vi "Configure Receiver Leveling Sweep Safe Mode.vi"(4 "Safe Mode Maximum Power Level (30)":dbl=30.0, 5 "Maximum Step Power Level (0)":dbl, 6 "Safe Mode Minimum Power Level (-200)":dbl=-200.0, 7 "Enable Safe Mode (F: Disabled)":bool, 8 "error in (no error)":errorcluster, 9 "Port ( 1)":i32=1, 10 "Channel (1)":i32=1, 11 "VISA resource name":refnum<visa-resource-name>) -> (0 "error out":errorcluster, 3 "VISA resource name out":refnum<visa-resource-name>)   [LabVIEW 2022 SP3, in "Agilent ENA Series.lvlib"]
doc: "Configures the receiver leveling information while in safe mode.\n\nNote:\nValid for E5072A only."
uses:
  Agilent ENA Series.lvlib
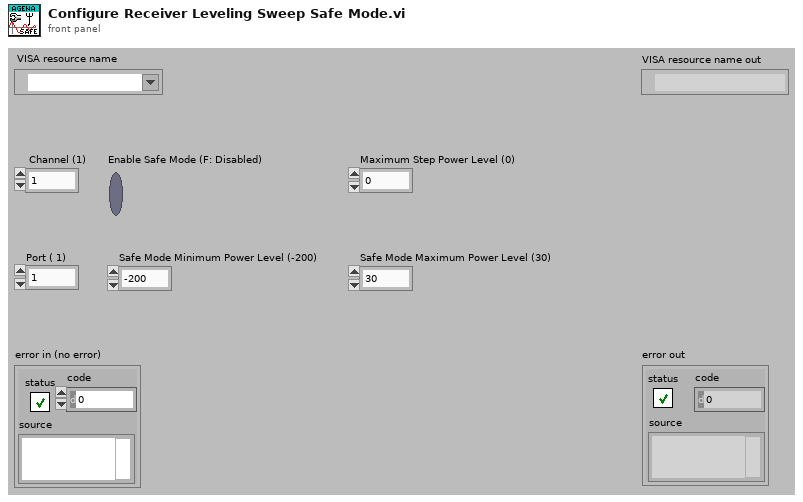
[diagram p1: front panel]
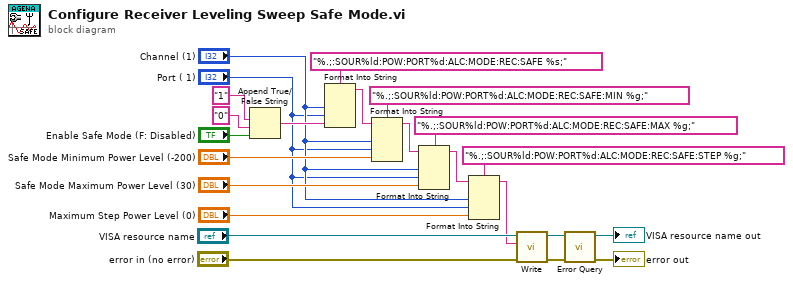
[diagram p0: block diagram]
diagram:
  n1 = Append True/False String(1:"Enable Safe Mode (F: Disabled)", 2:"0" ("false string"), 3:"1" ("true string")) -> (0:w16:string)  [unwired: 1 in]
  n2 = Format Into String(format string="%.;:SOUR%ld:POW:PORT%d:ALC:MODE:REC:SAFE %s;", "Channel (1)", "Port ( 1)", w16) -> (resulting string=w3:string)  [unwired: 2 in, 1 out]
  n3 = Format Into String(format string="%.;:SOUR%ld:POW:PORT%d:ALC:MODE:REC:SAFE:MIN %g;", initial string=w3, "Channel (1)", "Port ( 1)", "Safe Mode Minimum Power Level (-200)") -> (resulting string=w2:string)  [unwired: 1 in, 1 out]
  n4 = Format Into String(format string="%.;:SOUR%ld:POW:PORT%d:ALC:MODE:REC:SAFE:MAX %g;", initial string=w2, "Channel (1)", "Port ( 1)", "Safe Mode Maximum Power Level (30)") -> (resulting string=w4:string)  [unwired: 1 in, 1 out]
  n5 = Format Into String(format string="%.;:SOUR%ld:POW:PORT%d:ALC:MODE:REC:SAFE:STEP %g;", initial string=w4, "Channel (1)", "Port ( 1)", "Maximum Step Power Level (0)") -> (resulting string=w1:string)  [unwired: 1 in, 1 out]
  n6 = call "Write.vi"("error in (no error)"="error in (no error)", "String ()"=w1, "VISA resource name"="VISA resource name") -> ("error out"=w21:errorcluster, "VISA resource name out"=w20:refnum<visa-resource-name>)  [unwired: 6 in, 1 out]
  n7 = call "Error Query.vi"("error in (no error)"=w21, "VISA resource name"=w20) -> ("error out"=→"error out":errorcluster, "VISA resource name out"=→"VISA resource name out":refnum<visa-resource-name>)  [unwired: 6 in, 2 out]
